vi "2025_day9_Task01.vi"() -> ()   [LabVIEW 2025]
uses:
  <userlib>/_OpenG.lib/string/string.llb/openg_string.lvlib
panel:
  out "Task 1":i64
  in  "Switch":bool caption="Ex. Data  vs.  User Data"
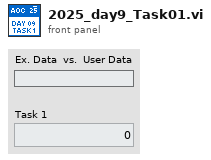
[diagram p1: front panel]
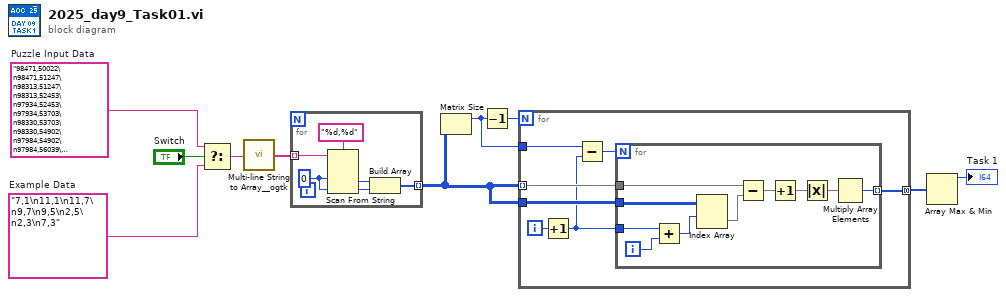
[diagram p0: block diagram]
diagram:
  w8 = "98471,50022\n98471,51247\n98313,51247\n98313,52453\n97934,52453\n97934,53703\n98330,53703\n98330,54902\n97984,54902\n97984,56039\n97240,56039\n97240,57357\n97876,57357\n97876,58495\n97270,58495\n97270,59614\n96671,59614\n96671,60903\n96888,60903\n96888,62000\n96259,62000\n96259,63234\n96170,63234\n96170,64294\n95484,64294\n95484,65695\n95847,65695\n95847,66844\n95416,66844\n95416,67945\n94865,67945\n94865,69031\n94291,69031\n94291,70224\n93962,70224\n93962,71368\n93511,71368\n93511,72053\n92171,72053\n92171,73477\n92251,73477\n92251,74151\n90983,74151\n90983,75481\n90838,75481\n90838,76375\n89979,76375\n89979,77664\n89706,77664\n89706,78338\n88553,78338\n88553,79457\n88019,79457\n88019,80302\n87127,80302\n87127,81267\n86387,81267\n86387,82151\n85553,82151\n85553,82744\n84414,82744\n84414,84022\n83990,84022\n83990,84817\n83065,84817\n83065,85878\n82384,85878\n82384,86344\n81171,86344\n81171,87168\n80277,87168\n80277,88118\n79477,88118\n79477,88556\n78284,88556\n78284,89226\n77275,89226\n77275,90211\n76474,90211\n76474,91032\n75548,91032\n75548,91563\n74440,91563\n74440,91909\n73235,91909\n73235,92811\n72337,92811\n72337,92991\n71063,92991\n71063,93616\n70015,93616\n70015,94542\n69090,94542\n69090,94639\n67806,94639\n67806,94846\n66585,94846\n66585,95789\n65627,95789\n65627,95571\n64274,95571\n64274,96029\n63147,96029\n63147,96763\n62084,96763\n62084,96559\n60781,96559\n60781,96836\n59602,96836\n59602,97680\n58522,97680\n58522,97154\n57201,97154\n57201,98028\n56093,98028\n56093,97593\n54817,97593\n54817,98354\n53659,98354\n53659,98323\n52427,98323\n52427,97524\n51181,97524\n51181,97846\n49977,97846\n49977,98297\n48753,98297\n48753,98068\n47539,98068\n47539,98323\n46297,98323\n46297,98240\n45071,98240\n45071,97608\n43913,97608\n43913,97725\n42665,97725\n42665,96813\n41586,96813\n41586,96817\n40355,96817\n40355,96378\n39214,96378\n39214,96924\n37826,96924\n37826,95702\n36899,95702\n36899,96091\n35514,96091\n35514,95597\n34390,95597\n34390,95239\n33220,95239\n33220,94779\n32088,94779\n32088,93884\n31143,93884\n31143,93180\n30135,93180\n30135,93044\n28860,93044\n28860,92455\n27797,92455\n27797,91649\n26857,91649\n26857,91247\n25692,91247\n25692,90376\n24806,90376\n24806,90415\n23336,90415\n23336,89589\n22417,89589\n22417,89029\n21311,89029\n21311,88010\n20549,88010\n20549,87143\n19684,87143\n19684,86505\n18631,86505\n18631,85541\n17859,85541\n17859,84916\n16777,84916\n16777,84156\n15810,84156\n15810,83265\n14971,83265\n14971,81923\n14632,81923\n14632,81552\n13211,81552\n13211,80350\n12742,80350\n12742,79451\n11915,79451\n11915,78583\n11036,78583\n11036,77631\n10261,77631\n10261,76316\n10028,76316\n10028,75266\n9421,75266\n9421,74433\n8448,74433\n8448,73500\n7613,73500\n7613,72300\n7259,72300\n7259,71253\n6619,71253\n6619,69845\n6753,69845\n6753,68970\n5735,68970\n5735,67618\n5831,67618\n5831,66479\n5438,66479\n5438,65382\n4927,65382\n4927,64295\n4363,64295\n4363,63235\n3662,63235\n3662,62049\n3373,62049\n3373,60900\n2924,60900\n2924,59725\n2561,59725\n2561,58416\n2911,58416\n2911,57199\n2858,57199\n2858,56048\n2329,56048\n2329,54825\n2322,54825\n2322,53621\n2148,53621\n2148,52432\n1579,52432\n1579,51184\n2388,51184\n2388,50020\n94646,50020\n94646,48765\n2174,48765\n2174,47554\n2231,47554\n2231,46301\n1727,46301\n1727,45164\n2674,45164\n2674,43939\n2593,43939\n2593,42738\n2746,42738\n2746,41592\n3216,41592\n3216,40270\n2766,40270\n2766,39223\n3658,39223\n3658,37939\n3510,37939\n3510,36720\n3671,36720\n3671,35628\n4269,35628\n4269,34473\n4645,34473\n4645,33455\n5393,33455\n5393,32043\n5107,32043\n5107,30931\n5621,30931\n5621,29737\n5955,29737\n5955,29028\n7296,29028\n7296,27650\n7262,27650\n7262,26477\n7666,26477\n7666,25726\n8808,25726\n8808,24690\n9437,24690\n9437,23306\n9538,23306\n9538,22671\n10775,22671\n10775,21468\n11183,21468\n11183,20509\n11938,20509\n11938,19899\n13119,19899\n13119,18489\n13329,18489\n13329,17994\n14608,17994\n14608,16802\n15109,16802\n15109,15883\n15915,15883\n15915,15538\n17272,15538\n17272,14439\n17902,14439\n17902,13668\n18840,13668\n18840,12580\n19517,12580\n19517,11863\n20508,11863\n20508,11260\n21581,11260\n21581,10882\n22800,10882\n22800,9793\n23529,9793\n23529,9029\n24489,9029\n24489,8441\n25562,8441\n25562,7944\n26683,7944\n26683,7208\n27673,7208\n27673,6563\n28718,6563\n28718,5925\n29774,5925\n29774,5545\n30947,5545\n30947,5535\n32262,5535\n32262,4757\n33268,4757\n33268,5035\n34654,5035\n34654,3762\n35516,3762\n35516,3727\n36783,3727\n36783,3055\n37868,3055\n37868,3000\n39116,3000\n39116,2784\n40319,2784\n40319,2650\n41536,2650\n41536,2542\n42752,2542\n42752,2662\n43993,2662\n43993,2022\n45143,2022\n45143,2463\n46402,2463\n46402,2277\n47602,2277\n47602,1831\n48801,1831\n48801,1998\n50022,1998\n50022,2190\n51234,2190\n51234,2218\n52445,2218\n52445,1831\n53690,1831\n53690,2570\n54845,2570\n54845,2167\n56114,2167\n56114,2300\n57330,2300\n57330,2295\n58573,2295\n58573,3449\n59589,3449\n59589,2860\n60962,2860\n60962,3739\n62000,3739\n62000,4162\n63139,4162\n63139,4059\n64437,4059\n64437,4412\n65606,4412\n65606,5182\n66622,5182\n66622,5010\n67995,5010\n67995,6186\n68826,6186\n68826,6383\n70065,6383\n70065,6698\n71265,6698\n71265,7546\n72201,7546\n72201,8307\n73166,8307\n73166,8429\n74497,8429\n74497,9624\n75192,9624\n75192,9652\n76618,9652\n76618,10416\n77578,10416\n77578,11497\n78300,11497\n78300,11714\n79663,11714\n79663,13191\n80041,13191\n80041,13642\n81241,13642\n81241,14248\n82330,14248\n82330,14963\n83335,14963\n83335,16367\n83664,16367\n83664,16716\n85047,16716\n85047,18088\n85354,18088\n85354,18629\n86576,18629\n86576,19482\n87462,19482\n87462,20562\n88066,20562\n88066,21712\n88559,21712\n88559,22716\n89239,22716\n89239,23785\n89816,23785\n89816,24399\n91114,24399\n91114,25707\n91310,25707\n91310,26664\n92088,26664\n92088,27862\n92429,27862\n92429,29056\n92747,29056\n92747,29953\n93682,29953\n93682,31166\n93943,31166\n93943,32079\n94924,32079\n94924,33522\n94555,33522\n94555,34553\n95260,34553\n95260,35724\n95573,35724\n95573,36725\n96474,36725\n96474,37952\n96621,37952\n96621,39072\n97189,39072\n97189,40437\n96643,40437\n96643,41485\n97631,41485\n97631,42735\n97567,42735\n97567,43928\n97855,43928\n97855,45151\n97902,45151\n97902,46394\n97641,46394\n97641,47601\n97746,47601\n97746,48807\n97933,48807\n97933,50022"  # Puzzle Input Data
  w9 = "7,1\n11,1\n11,7\n9,7\n9,5\n2,5\n2,3\n7,3"  # Example Data
  n1 = Select(t=w8, s="Switch", f=w9) -> (s? t:f=w7:string)
  n2 = call <userlib>:"Multi-line String to Array__ogtk.vi"("string"=w7) -> ("lines"=w6:string[])
  n3 = for {
    tunnel: w6 -> [w16] mode=indexing
    tunnel: [w12] -> w4 mode=indexing
    w11 = i64 0 ("default value 14")
    n4 = Scan From String(format string="%d,%d", input string=w16, default 1=w11, default 2=w11) -> (output 1=w14:i64, output 2=w13:i64)  [unwired: 2 in, 3 out]
    n5 = Build Array(w14, w13) -> (w12:i64[])
  }
  n6 = Matrix Size(0:w4) -> (1:w3:i32)  [unwired: 1 out]
  n7 = Decrement(x=w3) -> (x-1=w5:i32)
  n8 = for {
    N: w5 -> [_]
    tunnel: w4 -> [w22] mode=indexing
    tunnel: w4 -> [w21]
    tunnel: w3 -> [w19]
    tunnel: [w17] -> w2 mode=concatenating
    i -> [w23]
    n9 = Increment(x=w23) -> (x+1=w18:i32)
    n10 = Subtract(x=w19, y=w18) -> (x-y=w20:i32)
    n11 = for {
      N: w20 -> [_]
      tunnel: w18 -> [w33]
      tunnel: w22 -> [w26]
      tunnel: w21 -> [w30]
      tunnel: [w27] -> w17 mode=indexing
      i -> [w32]
      n12 = Add(x=w33, y=w32) -> (x+y=w31:i32)
      n13 = Index Array(array=w30, index (row)=w31) -> (element=w25:i64[])  [unwired: 1 in]
      n14 = Subtract(x=w26, y=w25) -> (x-y=w29:i64[])
      n15 = Increment(x=w29) -> (x+1=w24:i64[])
      n16 = Absolute Value(x=w24) -> (abs(x)=w28:i64[])
      n17 = Multiply Array Elements(1:w28) -> (0:w27:i64)
    }
  }
  n18 = Array Max & Min(array=w2) -> (max value=→"Task 1":i64)  [unwired: 3 out]
